vi "E441X_PM_Configure_Measurement.vi"(0 "VISA session":refnum<visa-resource-name>, 1 "Measurement (1)":i32=1, 5 "Measuring Function (0: Single)":i32(ring) items=["Single", "Single Relative", "Difference", "Difference Relative", "Ratio", "Ratio Relative"], 7 "Sensor 1 (0: Channel A)":i32(ring) items=["Channel A", "Channel B"], 9 "Sensor 2 (0: Channel A)":i32(ring) items=["Channel A", "Channel B"], 11 "error in (no error)":errorcluster {"code" format="%.0x"}, 12 "Resolution (3)":i32=3, 13 "Unit (0: dBm)":i32(ring) items=["dBm", "W"]) -> (4 "dup VISA session":refnum<visa-resource-name>, 15 "error out":errorcluster {"code" format="%.0x"})   [LabVIEW 2015]
doc: "This VI configures the measurement."
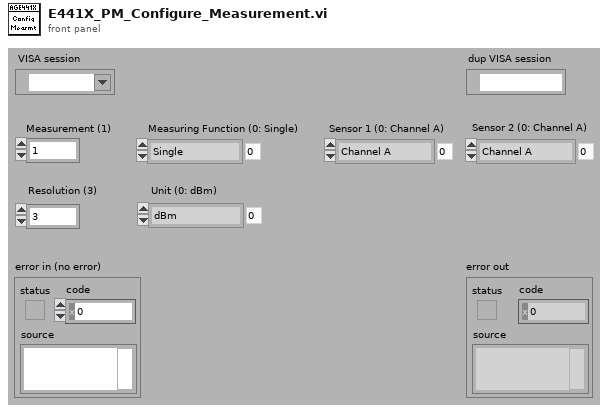
[diagram p1: front panel]
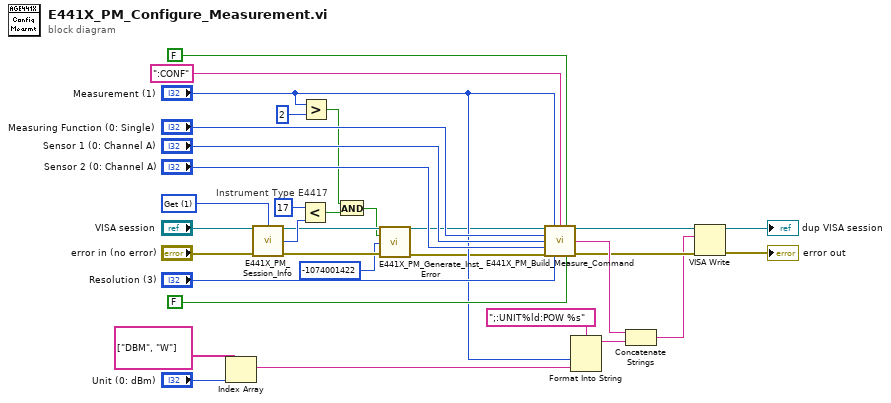
[diagram p0: block diagram]
diagram:
  w13 = 1 items=["Set", "Get"] ("Operation")
  # "Instrument Type E4417"
  n1 = Index Array(array=string[] ["DBM", "W"], index="Unit (0: dBm)") -> (element=w23:string)
  n2 = call "E441X_PM_Session_Info.vi"("VISA session"="VISA session", "Operation"=w13, "error in (no error)"="error in (no error)") -> ("dup VISA session"=w6:refnum<visa-resource-name>, "Instrument Number"=w12:i32, "error out"=w5:errorcluster)  [unwired: 7 in, 3 out]
  n3 = Less?(x=17, y=w12) -> (x < y?=w10:bool)
  n4 = Greater?(x="Measurement (1)", y=2 ("x")) -> (0:w7:bool)
  n5 = And(x=w7, y=w10) -> (x .and. y?=w4:bool)
  n6 = call "E441X_PM_Generate_Inst_Error.vi"("VISA session"=w6, "Error State (F: Off)"=w4, "Code (0 - No error)"=-1074001422, "error in (no error)"=w5) -> ("dup VISA session"=w2:refnum<visa-resource-name>, "error out"=w3:errorcluster)  [unwired: 10 in]
  n7 = call "E441X_PM_Build_Measure_Command.vi"("VISA session"=w2, "Measurement (1)"="Measurement (1)", "Command"=":CONF", "Question (F: No Question)"=FALSE, "Measuring Function (0: Single)"="Measuring Function (0: Single)", "Sensor 1 (0: Channel A)"="Sensor 1 (0: Channel A)", "Sensor 2 (0: Channel A)"="Sensor 2 (0: Channel A)", "error in (no error)"=w3, "Resolution (3)"="Resolution (3)", "Expected Value (F: Off)"=FALSE ("Question (F: No Question)")) -> ("dup VISA session"=w19:refnum<visa-resource-name>, "Output Command"=w21:string, "error out"=w18:errorcluster)  [unwired: 3 in]
  n8 = Format Into String(format string=";:UNIT%ld:POW %s", "Measurement (1)", w23) -> (resulting string=w22:string)  [unwired: 2 in, 1 out]
  n9 = Concatenate Strings(w21, w22) -> (w17:string)
  n10 = VISA Write(VISA resource name=w19, write buffer=w17, error in (no error)=w18) -> (VISA resource name out=→"dup VISA session":refnum<visa-resource-name>, error out=→"error out":errorcluster)  [unwired: 1 out]
